vi "SA_LitePoint_RS.vi"() -> ()   [LabVIEW 2023]
uses:
  CTL/LitePoint_EVM_SA.ctl
  R_S/R_S.lvlib
  LitePoints/LitePoints.lvlib
panel:
  out "error out":errorcluster
  in  "error in":errorcluster
  in  "VISA IN":refnum<visa-resource-name>="IQGIG"
  in  "Function":enum16{"Initilize", "getPower", "Close"}(ring)
  in  "Equipment?":enum16{"Litepoint", "R&S"}(ring)
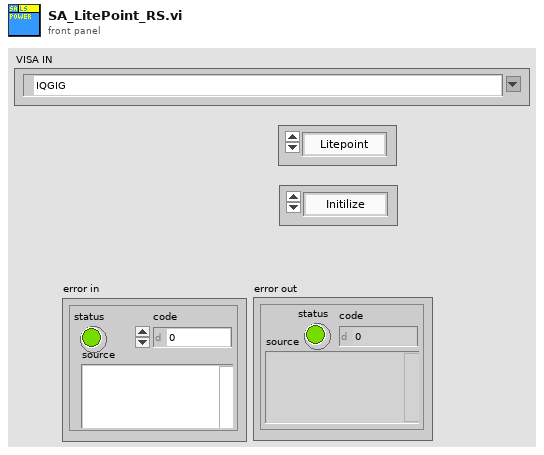
[diagram p1: front panel]
types:
  T1 = typedef "LitePoint_EVM_SA.ctl" = enum16{"Init", "Close", "set_SA", "get_EVM", "byPass", "getPower"}
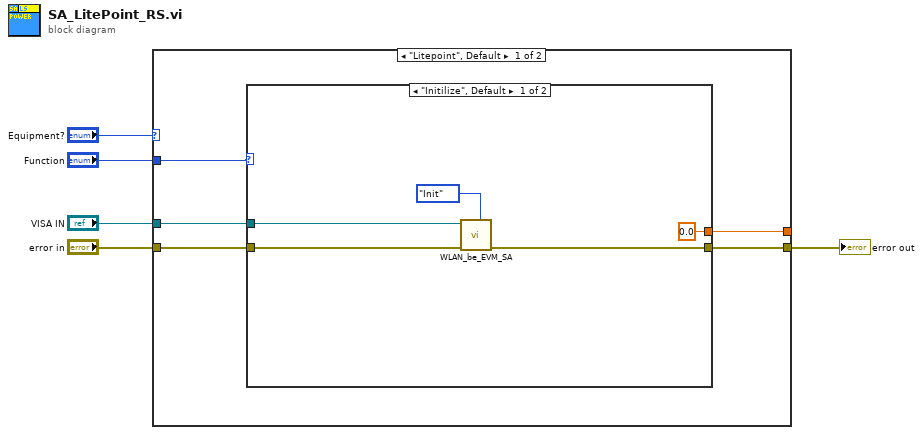
[diagram p0: block diagram]
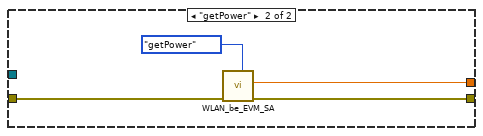
[diagram p2: hidden frame]
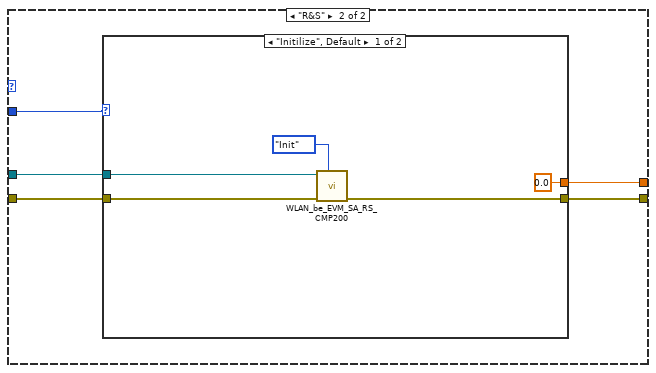
[diagram p3: hidden frame]
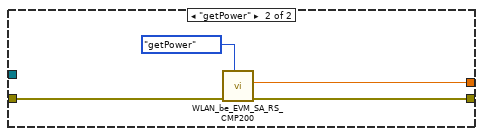
[diagram p4: hidden frame]
diagram:
  n1 = case shown="\"Litepoint\", Default" "Equipment?" {
    tunnel: "Function" -> [w10 w24]
    tunnel: "VISA IN" -> [w9 w23]
    tunnel: "error in" -> [w8 w22]
    tunnel: [w7 w21] -> w1
    tunnel: [w6 w20] -> _
    frame "Litepoint", Default {
      n2 = case shown="\"Initilize\", Default" w10 {
        tunnel: w9 -> [w15 _]
        tunnel: w8 -> [w14 w19]
        tunnel: [w13 w18] -> w7
        tunnel: [0.0 ("Power") w16] -> w6
        frame "Initilize", Default {
          n3 = call "WLAN_be_EVM_SA.vi"("Function"=LitePoint_EVM_SA."Init", "error in"=w14, "VISA IN"=w15) -> ("error out"=w13:errorcluster)  [unwired: 5 in, 3 out]
        }
        frame "getPower" {
          n4 = call "WLAN_be_EVM_SA.vi"("Function"=LitePoint_EVM_SA."getPower", "error in"=w19) -> ("error out"=w18:errorcluster, "Power"=w16:dbl)  [unwired: 6 in, 2 out]
        }
      }
    }
    frame "R&S" {
      n5 = case shown="\"Initilize\", Default" w24 {
        tunnel: w23 -> [w29 _]
        tunnel: w22 -> [w28 w33]
        tunnel: [w27 w32] -> w21
        tunnel: [0.0 ("Power") w30] -> w20
        frame "Initilize", Default {
          n6 = call "WLAN_be_EVM_SA_RS_CMP200.vi"("Function"=LitePoint_EVM_SA."Init", "error in"=w28, "VISA IN"=w29) -> ("error out"=w27:errorcluster)  [unwired: 5 in, 3 out]
        }
        frame "getPower" {
          n7 = call "WLAN_be_EVM_SA_RS_CMP200.vi"("Function"=LitePoint_EVM_SA."getPower", "error in"=w33) -> ("error out"=w32:errorcluster, "Power"=w30:dbl)  [unwired: 6 in, 2 out]
        }
      }
    }
  }
  "error out" <- w1
